vi "Uninit.vi"(2 "Container State":T1, 3 "Display State":T2) -> ()   [LabVIEW 2020, in "3D Surface.xctl"]
uses:
  <vilib>/Math Plots/3D Math Plots/3D Surface/3D Surface XCtrl/3D Surface.xctl
  <vilib>/Math Plots/3D Math Plots/3D Surface/3D Surface XCtrl/State.ctl
  <vilib>/Math Plots/3D Math Plots/3D Surface/3D Surface/3D Surface.lvclass
  <vilib>/Math Plots/3D Math Plots/3D Plot/Action String/3DMathPlot Ctrl Act Queue.ctl
  <vilib>/Math Plots/3D Math Plots/3D Plot/Action String/3DMathPlot Ctrl Act Cluster.ctl
  <vilib>/Math Plots/3D Math Plots/3D Plot/Action String/3DMathPlot State Class.ctl
  <vilib>/_xctls/Container State.ctl
  <vilib>/_xctls/XControlSupport.lvlib
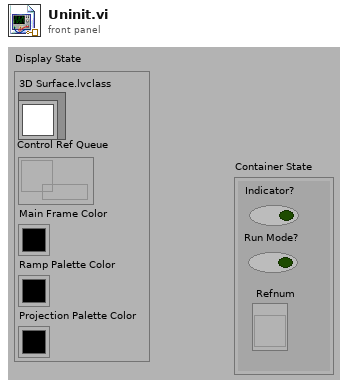
[diagram p1: front panel]
types:
  T1 = typedef "XControlSupport.lvlib/Container State.ctl" = cluster{"Indicator?":bool, "Run Mode?":bool, " Refnum":refnum<vi>}
  T2 = typedef "3D Surface.xctl/State.ctl" = cluster{"3D Surface.lvclass":refnum<class "3D Surface.lvclass">, "Control Ref Queue":T3, "Main Frame Color":u32, "Ramp Palette Color":u32, "Projection Palette Color":u32}
  T3 = typedef "3DMathPlot Ctrl Act Queue.ctl" = refnum<queue>
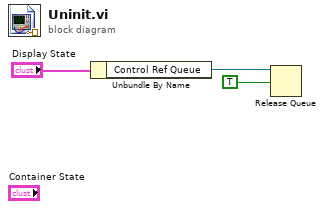
[diagram p0: block diagram]
diagram:
  n1 = Unbundle By Name("Display State") -> ("Control Ref Queue"=w2:T3)
  n2 = Release Queue(queue=w2, force destroy? (F)=TRUE) -> ()  [unwired: 1 in, 3 out]
